vi "products.vi"(8 "error in (no error)":errorcluster, 11 "reference in":refnum<class "Project Panels.lvclass">=refnum) -> (0 "error out":errorcluster, 3 "reference out":refnum<class "Project Panels.lvclass">)   [LabVIEW 2015, in "Project Panels.lvclass"]
uses:
  Project Panels.lvclass
  state.ctl
  <vilib>/Utility/miscctls.llb/LVRowAndColumnUnsignedTypeDef.ctl
  SYS/Devices Controller_llb/deviceType.ctl
  <vilib>/Utility/miscctls.llb/LVRowAndColumnTypeDef.ctl
  SYS/Devices Controller_llb/Devices Controller.lvclass
panel:
  out "title":string="Cosmed Asia Pacific - Products in Aussie"
  in  "tables":T1(tab)
  out "K5":string[][](table)=[["705001", "not active", "K4b2", "not active", "not active", "not active", "not active", "not active", "not active", "not active", "not active", "not active", ""], ["803033", "not active", "K4b2", "not active", "not active", "not active", "not active", "not active", "not active", "not active", "not active", "not active", ""], ["804042", "not active", "K4b2", "not active", "not active", "not active", "not active", "not active", "not active", "not active", "not active", "not active", ""], ["804046", "", "K4b2", "Univ. of Queensland", "St Lucia, Brisbane", "Gary Wilson", "seant@hms.uq.edu.au", "Bellamby", "sep-06", "Italy", "sep-07", "not active", ""], ["804047", "not active", "K4b2", "not active", "not active", "not active", "not active", "not active", "not active", "not active", "not active", "not active", ""], ["9806059", "6.2", "K4b2", "not active", "not active", "not active", "not active", "not active", "not active", "not active", "not active", "not active", ""], ["9806062", "5.1", "K4b2", "Queensland Academy of Sport", "Sunnybank", "Mark Andrews", "mark.andrews@srq.qld.com.au", "Nahtan, GC", "june 2013 in italy for CO2 refurbish", "Italy service", "jun-14", "", ""], ["9807077", "6.0a", "K4b2", "Uni of Canterbury", "Uni of Canterbury", "Gavin Blackwell", "gavin.blackwell@canterbury.ac.nz", "Christchurch", "feb-13", "fede", "feb-14", "", ""], ["9810080", "", "K4b2", "Royal Children's Hospital", "Herston", "Teresa Phillips", "Teresa_Phillips@health.qld.gov.au", "Herston", "jun-06", "Italy", "jun-07", "9/17/2013", ""], ["9903123", "7.2", "K4b2", "Uni of Adelaide", "Uni of Adelaide", "David Bentley", "david.bentley@adelaide.edu.au", "Adelaide", "dic-12", "Serv Italy +valve", "dic-13", "", ""], ["9912206", "7.3", "K4b2", "Uni of Canterbury", "Uni of Canterbury", "Gavin Blackwell", "gavin.blackwell@canterbury.ac.nz", "Christchurch", "feb-13", "fede", "feb-14", "", ""], ["200104325", "8", "K4b2", "Uni of South Australia", "Sansom Institute", "Michelle N. McDonnell", "", "Adelaide", "nov-11", "fede", "dic-12", "9/9/2013", ""], ["200201385", "9.1b", "K4b2", "University of Sydney", "Lidcombe Campus", "Hui Yin Ler  (PhD)", "", "Sydney", "oct-11", "fede", "oct-12", "9/9/2013", ""], ["200205419", "8.0", "K4b2", "University of Sydney", "Liverpool hospital", "Leanne Hassett", "leanne.hassett@sydney.edu.au", "Sydney", "nov-11", "fede", "nov-12", "Not Using in this moment", ""], ["200205423", "9.1b", "K4b2", "University of Sydney", "Lidcombe Campus", "Martin Thomson", "", "Sydney", "feb-10", "italy", "feb-11", "9/9/2013", ""], ["200205424", "7.3", "K4b2", "University of Sydney", "Lidcombe Campus", "Martin Thomson", "", "Sydney", "sep-08", "Italy", "sep-09", "9/10/2013", ""], ["200404607", "", "K4b2", "The Sydney Children's Hospital Network", "Westmead", "Leanne Purcell", "leanne.purcell@health.nsw.gov.au", "Westmead", "nov-08", "italy", "nov-09", "9/17/2013", "Yes, but waiting the start of the testing"], ["200512701", "8.0b", "K4b2", "James Cook Uni", "James Cook Uni", "Anthony Leight", "Anthony.Leicht@jcu.edu.au", "Townsville", "jan-13", "", "jan-14", "", ""], ["200601705", "", "K4b2", "Latrobe University", "Bundoora (Melb)", "Paul Moon", "P.Moon@latrobe.edu.au", "Melbourne", "jan-08", "Italy", "jan-09", "9/17/2013", ""], ["200607745", "", "K4b2", "QUT Brisbane", "Kelvin Grove", "Pei Cher", "pei.cher@qut.edu.au", "BBN", "may-13", "fede", "may-14", "", ""], ["200710813", "", "K4b2", "Victoria Uni", "", "Jessica Meilak", "jessica.meilak@vu.edu.au", "Melb", "jan-12", "Brad", "jan-14", "15/01/14", ""], ["200907909", "9.1b", "K4b2", "Uni of New South Wales", "Uni of New South Wales", "Stephen Redmond", "s.redmond@unsw.edu.au", "Sydney", "sep-12", "fede", "sep-13", "9/17/2013", ""], ["200909916", "", "K4b2", "Uni of Canterbury", "Uni of Canterbury", "Gavin Blackwell", "gavin.blackwell@canterbury.ac.nz", "Christchurch", "feb-13", "fede", "feb-14", "", ""], ["201007964", "", "K4b2", "University of Canberra", "Canberra", "Ben Rattray", "ben.rattray@canberra.edu.au", "Canberra", "mar-12", "", "mar-13", "9/17/2013", ""], ["201009980", "9.1b", "K4b2", "Uni of Technology Sydney", "UTS City Campus", "Steven Su", "steven.su@eng.uts.edu.au", "Sydney", "oct-12", "Medtel (also Lee Valve)", "oct-13", "9/17/2013", ""], ["2011121063", "", "K4b2", "Victoria Uni", "", "Jessica Meilak", "jessica.meilak@vu.edu.au", "Melb", "jan-12", "Brad", "jan-14", "", ""], ["2011121064", "", "K4b2", "Victoria Uni", "", "Jessica Meilak", "jessica.meilak@vu.edu.au", "Melb", "jan-12", "Brad", "jan-14", "", ""], ["2012021076", "", "K4b2", "Demo Unit", "Demo Unit", "TBD", "", "TBD", "sep-13", "Manu-AUS", "sep-14", "", ""], ["2012021080", "", "K4b2", "Massey Univ.", "Wellington", "Brandon Woolley", "B.Woolley@massey.ac.nz", "Wellington", "nov-13", "Manu-AUS", "nov-14", "", ""], ["2012061109", "", "K4b2", "Griffith University Gold Coast Campus", "Gold Coast", "Anna Boehm", "a.boehm@griffith.edu.au", "Gold Coast", "jul-13", "fede", "jul-14", "", ""], ["2012061115", "10.0d", "K4b2", "University of Newcastle", "Callaghan", "Robin Callister", "Robin.Callister@newcastle.edu.au", "Ourimbah", "nov-13", "Manu-AUS", "nov-14", "", ""], ["2012111144", "10.0d", "K4b2", "University of Newcastle", "Callaghan", "Robin Callister", "Robin.Callister@newcastle.edu.au", "Ourimbah", "nov-13", "Manu-AUS", "nov-14", "", ""], ["2012111148", "", "K4b2", "University of Western Sydney", "PENRITH", "Tara Hamilton", "t.hamilton@uws.edu.au", "PENRITH", "dec-13", "Manu-AUS", "dec-14", "", ""], ["2013011158", "10.0d", "K4b2", "University of the Sunshine Coast", "Maroochydore DC", "Ava Kerr", "akerr@usc.edu.au", "Sippy Downs", "may-13", "new", "may-14", "", ""], ["2013031168", "10.0d", "K4b2", "Australian Catholic University", "Sydney", "Phillip Chapman", "Phillip.Chapman@acu.edu.au", "Sydney", "apr-13", "new", "apr-14", "", ""], ["Prova", "", "Prova", "", "", "", "", "", "", "", "", "", ""]]
  out "k4b2":string[][](table)=[["705001", "not active", "K4b2", "not active", "not active", "not active", "not active", "not active", "not active", "not active", "not active", "not active", ""], ["803033", "not active", "K4b2", "not active", "not active", "not active", "not active", "not active", "not active", "not active", "not active", "not active", ""], ["804042", "not active", "K4b2", "not active", "not active", "not active", "not active", "not active", "not active", "not active", "not active", "not active", ""], ["804046", "", "K4b2", "Univ. of Queensland", "St Lucia, Brisbane", "Gary Wilson", "seant@hms.uq.edu.au", "Bellamby", "sep-06", "Italy", "sep-07", "not active", ""], ["804047", "not active", "K4b2", "not active", "not active", "not active", "not active", "not active", "not active", "not active", "not active", "not active", ""], ["9806059", "6.2", "K4b2", "not active", "not active", "not active", "not active", "not active", "not active", "not active", "not active", "not active", ""], ["9806062", "5.1", "K4b2", "Queensland Academy of Sport", "Sunnybank", "Mark Andrews", "mark.andrews@srq.qld.com.au", "Nahtan, GC", "june 2013 in italy for CO2 refurbish", "Italy service", "jun-14", "", ""], ["9807077", "6.0a", "K4b2", "Uni of Canterbury", "Uni of Canterbury", "Gavin Blackwell", "gavin.blackwell@canterbury.ac.nz", "Christchurch", "feb-13", "fede", "feb-14", "", ""], ["9810080", "", "K4b2", "Royal Children's Hospital", "Herston", "Teresa Phillips", "Teresa_Phillips@health.qld.gov.au", "Herston", "jun-06", "Italy", "jun-07", "9/17/2013", ""], ["9903123", "7.2", "K4b2", "Uni of Adelaide", "Uni of Adelaide", "David Bentley", "david.bentley@adelaide.edu.au", "Adelaide", "dic-12", "Serv Italy +valve", "dic-13", "", ""], ["9912206", "7.3", "K4b2", "Uni of Canterbury", "Uni of Canterbury", "Gavin Blackwell", "gavin.blackwell@canterbury.ac.nz", "Christchurch", "feb-13", "fede", "feb-14", "", ""], ["200104325", "8", "K4b2", "Uni of South Australia", "Sansom Institute", "Michelle N. McDonnell", "", "Adelaide", "nov-11", "fede", "dic-12", "9/9/2013", ""], ["200201385", "9.1b", "K4b2", "University of Sydney", "Lidcombe Campus", "Hui Yin Ler  (PhD)", "", "Sydney", "oct-11", "fede", "oct-12", "9/9/2013", ""], ["200205419", "8.0", "K4b2", "University of Sydney", "Liverpool hospital", "Leanne Hassett", "leanne.hassett@sydney.edu.au", "Sydney", "nov-11", "fede", "nov-12", "Not Using in this moment", ""], ["200205423", "9.1b", "K4b2", "University of Sydney", "Lidcombe Campus", "Martin Thomson", "", "Sydney", "feb-10", "italy", "feb-11", "9/9/2013", ""], ["200205424", "7.3", "K4b2", "University of Sydney", "Lidcombe Campus", "Martin Thomson", "", "Sydney", "sep-08", "Italy", "sep-09", "9/10/2013", ""], ["200404607", "", "K4b2", "The Sydney Children's Hospital Network", "Westmead", "Leanne Purcell", "leanne.purcell@health.nsw.gov.au", "Westmead", "nov-08", "italy", "nov-09", "9/17/2013", "Yes, but waiting the start of the testing"], ["200512701", "8.0b", "K4b2", "James Cook Uni", "James Cook Uni", "Anthony Leight", "Anthony.Leicht@jcu.edu.au", "Townsville", "jan-13", "", "jan-14", "", ""], ["200601705", "", "K4b2", "Latrobe University", "Bundoora (Melb)", "Paul Moon", "P.Moon@latrobe.edu.au", "Melbourne", "jan-08", "Italy", "jan-09", "9/17/2013", ""], ["200607745", "", "K4b2", "QUT Brisbane", "Kelvin Grove", "Pei Cher", "pei.cher@qut.edu.au", "BBN", "may-13", "fede", "may-14", "", ""], ["200710813", "", "K4b2", "Victoria Uni", "", "Jessica Meilak", "jessica.meilak@vu.edu.au", "Melb", "jan-12", "Brad", "jan-14", "15/01/14", ""], ["200907909", "9.1b", "K4b2", "Uni of New South Wales", "Uni of New South Wales", "Stephen Redmond", "s.redmond@unsw.edu.au", "Sydney", "sep-12", "fede", "sep-13", "9/17/2013", ""], ["200909916", "", "K4b2", "Uni of Canterbury", "Uni of Canterbury", "Gavin Blackwell", "gavin.blackwell@canterbury.ac.nz", "Christchurch", "feb-13", "fede", "feb-14", "", ""], ["201007964", "", "K4b2", "University of Canberra", "Canberra", "Ben Rattray", "ben.rattray@canberra.edu.au", "Canberra", "mar-12", "", "mar-13", "9/17/2013", ""], ["201009980", "9.1b", "K4b2", "Uni of Technology Sydney", "UTS City Campus", "Steven Su", "steven.su@eng.uts.edu.au", "Sydney", "oct-12", "Medtel (also Lee Valve)", "oct-13", "9/17/2013", ""], ["2011121063", "", "K4b2", "Victoria Uni", "", "Jessica Meilak", "jessica.meilak@vu.edu.au", "Melb", "jan-12", "Brad", "jan-14", "", ""], ["2011121064", "", "K4b2", "Victoria Uni", "", "Jessica Meilak", "jessica.meilak@vu.edu.au", "Melb", "jan-12", "Brad", "jan-14", "", ""], ["2012021076", "", "K4b2", "Demo Unit", "Demo Unit", "TBD", "", "TBD", "sep-13", "Manu-AUS", "sep-14", "", ""], ["2012021080", "", "K4b2", "Massey Univ.", "Wellington", "Brandon Woolley", "B.Woolley@massey.ac.nz", "Wellington", "nov-13", "Manu-AUS", "nov-14", "", ""], ["2012061109", "", "K4b2", "Griffith University Gold Coast Campus", "Gold Coast", "Anna Boehm", "a.boehm@griffith.edu.au", "Gold Coast", "jul-13", "fede", "jul-14", "", ""], ["2012061115", "10.0d", "K4b2", "University of Newcastle", "Callaghan", "Robin Callister", "Robin.Callister@newcastle.edu.au", "Ourimbah", "nov-13", "Manu-AUS", "nov-14", "", ""], ["2012111144", "10.0d", "K4b2", "University of Newcastle", "Callaghan", "Robin Callister", "Robin.Callister@newcastle.edu.au", "Ourimbah", "nov-13", "Manu-AUS", "nov-14", "", ""], ["2012111148", "", "K4b2", "University of Western Sydney", "PENRITH", "Tara Hamilton", "t.hamilton@uws.edu.au", "PENRITH", "dec-13", "Manu-AUS", "dec-14", "", ""], ["2013011158", "10.0d", "K4b2", "University of the Sunshine Coast", "Maroochydore DC", "Ava Kerr", "akerr@usc.edu.au", "Sippy Downs", "may-13", "new", "may-14", "", ""], ["2013031168", "10.0d", "K4b2", "Australian Catholic University", "Sydney", "Phillip Chapman", "Phillip.Chapman@acu.edu.au", "Sydney", "apr-13", "new", "apr-14", "", ""], ["Prova", "", "Prova", "", "", "", "", "", "", "", "", "", ""]]
  out "fitmate":string[][](table)=[["2005090013", "2.2", "Fitmate Pro", "Wesley Weight Management", "Milton", "Liz Ernst", "eernst@lifeshape.com.au", "Milton", "27/09", ""], ["2006020058", "1", "Fitmate WM", "Toombul Medical Centre", "Spring Hill", "Zoe Glover", "toombulmc@gmail.com", "Spring Hill", "27/09", ""], ["2006020059", "1", "Fitmate WM", "RMIT Univ.", "Melbourne", "George Lenon", "george.lenon@rmit.edu.au", "Melbourne", "27/09", ""], ["2006020060", "1", "Fitmate WM", "Logan Hospital", "Meadowbrook", "??", "??", "Meadowbrook", "", ""], ["2006020061", "1.6", "Fitmate WM", "Biomedex (Aust) Pty Ltd", "Woonona", "Biomedex (Aust) Pty Ltd", "??", "Woonona", "", ""], ["2006020077", "1", "Fitmate Pro", "Wesley Weight Management", "Southport", "Sally Jordan", "SJordan@weshealth.com.au", "Southport", "27/09 mail come back / no problem", ""], ["2006020078", "1", "Fitmate Pro", "Life4Ever Pty Ltd", "Arundel", "Michael Tait", "mail@drmichaeltait.com", "Arundel", "27/09 mail come back", ""], ["2006030062", "2.2", "Fitmate WM", "Biomedex (Aust) Pty Ltd", "Woonona", "Biomedex (Aust) Pty Ltd", "??", "Woonona", "", ""], ["2006030083", "2", "Fitmate Pro", "Australian College of Physical Education", "Olympic Park Sydney", "Sven Rees", "srees@acpe.edu.au", "Olympic Park Sydney", "30/09", ""], ["2006030084", "2.3", "Fitmate Pro", "Monash Univ. The Alfred Centre", "Frankston", "Tim Wallace", "tim.wallace@monash.edu", "Frankston", "Case Opned for Macro error", ""], ["2006030085", "2.2", "Fitmate Pro", "Southside Exercise Therapy", "Gymea", "Luke Delvecchio", "southsidepty@optusnet.com.au", "Gymea", "30/09", ""], ["2006060076", "1.1", "Fitmate WM", "Edith Cowan Univ.", "Joondalup", "Amanda Devine", "a.devine@ecu.edu.au", "Joondalup", "30/09", ""], ["2006060078", "1.1", "Fitmate WM", "Edith Cowan Univ.", "Joondalup", "Amanda Devine", "a.devine@ecu.edu.au", "Joondalup", "30/09", ""], ["2006060080", "2.3", "Fitmate WM", "WESLEY Corporate Health", "Brisbane", "Liz Ernst", "eernst@lifeshape.com.au", "Brisbane", "27/09", ""], ["2006080185", "1.1", "Fitmate Pro", "Edith Cowan Univ.", "Joondalup", "Doreen Mackie", "DMackie@hotmail.com", "Joondalup", "Waiting for details from email (n.vrdoljak@ecu.edu.au   )", ""], ["2006080186", "1.1", "Fitmate Pro", "Neocardia PTY LTD", "Noosaville", "Neavison", "Neavison@hotmail.com", "Noosaville", "30/09", ""], ["2006080187", "1.1", "Fitmate Pro", "Kams Health and Fitness", "Armidale", "Kamahl Barhoush", "info@kams.com.au", "Armidale", "doesn't answer/call again", ""], ["2006080188", "1.1", "Fitmate Pro", "Edith Cowan Univ.", "Joondalup", "Doreen Mackie", "DMackie@hotmail.com", "Joondalup", "Waiting for details from email (n.vrdoljak@ecu.edu.au   )", ""], ["2006080189", "1.1", "Fitmate Pro", "Get Back On Track", "Victoria", "Lisa Ham", "LisaH@bigpond.com.au", "Victoria", "doesn't answer/call again", ""], ["2006080190", "1.1", "Fitmate Pro", "Edith Cowan Univ.", "Joondalup", "Doreen Mackie", "DMackie@hotmail.com", "Joondalup", "Waiting for details from email (n.vrdoljak@ecu.edu.au   )", ""], ["2006080191", "1.1", "Fitmate Pro", "One Life", "PADDINGTON", "Justin Lang", "admin@onelifeliveit.net.au", "PADDINGTON", "01/10", "NOT ACTIVE"], ["2007030363", "1.1", "Fitmate Pro", "X-Fitness Systems Ltd", "Auckland,", "Scott Tibbutt", "scott@xfitness.co.nz", "Auckland,", "30/09", ""], ["2007030372", "1.1", "Fitmate Pro", "Edith Cowan Univ.", "Joondalup", "Doreen Mackie", "DMackie@hotmail.com", "Joondalup", "Waiting for details from email (n.vrdoljak@ecu.edu.au   )", ""], ["2007030373", "1.1", "Fitmate Pro", "Edith Cowan Univ.", "Joondalup", "Doreen Mackie", "DMackie@hotmail.com", "Joondalup", "Waiting for details from email (n.vrdoljak@ecu.edu.au   )", ""], ["2007030375", "1.1", "Fitmate Pro", "Vision Health and Fitness", "Toowoomba", "Troy Taylor", "troy@visionhealth.com.au", "Toowoomba", "30/09", ""], ["2007050155", "2", "Fitmate WM", "Fitness Fusion", "Ohope", "Erin Baker", "paul@fitnessfusion.co.nz", "Ohope", "30/09", ""], ["2007050156", "1.1", "Fitmate WM", "X-Fitness Systems Ltd", "Auckland,", "X-Fitness Systems Ltd", "jeremyu@uhl.co.nz", "Auckland,", "30/09", ""], ["2007050157", "2.2", "Fitmate WM", "Wesley Weight Management", "Milton", "Liz Ernst", "eernst@lifeshape.com.au", "Milton", "27/09", ""], ["2007050158", "2.2", "Fitmate WM", "WESLEY Corporate Health", "Brisbane", "Liz Ernst", "eernst@lifeshape.com.au", "Brisbane", "27/09", ""], ["2007050159", "1.1", "Fitmate WM", "Wesley Weight Management", "Rockhampton", "Simon Fawssett", "sfawssett@weshealth.com.au", "Rockhampton", "no problem", ""], ["2007050160", "2.2", "Fitmate WM", "WESLEY Corporate Health", "Brisbane", "Liz Ernst", "eernst@lifeshape.com.au", "Brisbane", "27/09", ""], ["2007050161", "1.1", "Fitmate WM", "Pyrmont Health & Fitness Club", "Pyrmont", "Antoine Poulter", "??", "Pyrmont", "", ""], ["2007050376", "1.1", "Fitmate Pro", "Edith Cowan Univ.", "Joondalup", "Doreen Mackie", "DMackie@hotmail.com", "Joondalup", "Waiting for details from email (n.vrdoljak@ecu.edu.au   )", ""], ["2007050377", "1.1", "Fitmate Pro", "Elgin Street Medical Centre", "Carlton", "Daniel Cobb", "dcobb@live.com.au", "Carlton", "30/09", ""], ["2007050378", "1.1", "Fitmate Pro", "Pyrmont Health & Fitness Club", "Pyrmont", "Justine Justine", "??", "Pyrmont", "", ""], ["2007050379", "1.6", "Fitmate Pro", "HERT", "Millers Point", "Mark Newton", "mark@hert.com.au", "Millers Point", "30/09", ""], ["2007050380", "1.1", "Fitmate Pro", "Edith Cowan Univ.", "Joondalup", "Doreen Mackie", "DMackie@hotmail.com", "Joondalup", "Waiting for details from email (n.vrdoljak@ecu.edu.au   )", ""], ["2007050381", "1.6", "Fitmate Pro", "Fitness Development Australia", "Sydney", "Fitness Development Australia", "zarko_mikulic@hotmail.com", "Sydney", "30/09", ""], ["2007050388", "1.1", "Fitmate Pro", "ULO Pty Ltd", "Roebourne Court", "Adam Brown", "adam@ulo.com.au", "Daisy Hill", "30/09", ""], ["2007050395", "1.6", "Fitmate Pro", "Biomedex (Aust) Pty Ltd", "Woonona", "Biomedex (Aust) Pty Ltd", "??", "Woonona", "", ""], ["2007050404", "1.1", "Fitmate Pro", "Biomedex (Aust) Pty Ltd", "Woonona", "Biomedex (Aust) Pty Ltd", "??", "Woonona", "", ""], ["2007060413", "2", "Fitmate Pro", "Biomedex (Aust) Pty Ltd", "Woonona", "Biomedex (Aust) Pty Ltd", "??", "Woonona", "", ""], ["2007060415", "1.1", "Fitmate Pro", "Mater Childrens Hospital", "South Brisbane", "Gary Leong", "gary.leong@mater.org.au", "South Brisbane", "1/10/2013", ""], ["2007060417", "1.1", "Fitmate Pro", "Ray Kelly Fitness", "Blacktown", "Ray Kelly", "maxvel01@hotmail.com", "Blacktown", "30/09", ""], ["2007100277", "2.2", "Fitmate WM", "Biomedex (Aust) Pty Ltd", "Woonona", "Biomedex (Aust) Pty Ltd", "??", "Woonona", "", ""], ["2007100278", "1.1", "Fitmate WM", "Tone Up Weight Loss", "Campbelltown", "Christopher Satara", "scott@swphysio.com.au'", "Campbelltown", "08/10", ""], ["2007100279", "1.6", "Fitmate WM", "Biomedex (Aust) Pty Ltd", "Woonona", "Biomedex (Aust) Pty Ltd", "??", "Woonona", "", ""], ["2007100281", "2.2", "Fitmate WM", "Biomedex (Aust) Pty Ltd", "Woonona", "Biomedex (Aust) Pty Ltd", "??", "Woonona", "", ""], ["2007100282", "2.2", "Fitmate WM", "Biomedex (Aust) Pty Ltd", "Woonona", "Biomedex (Aust) Pty Ltd", "??", "Woonona", "", ""], ["2007100484", "2.3", "Fitmate Pro", "Univ. of Auckland", "Auckland", "Grant Mawston", "", "Auckland", "", ""], ["2008010568", "2.3", "Fitmate Pro", "Australian College of", "Olympic Park Sydney", "Sven Rees", "srees@acpe.edu.au", "Olympic Park Sydney", "30/09", ""], ["2008010576", "2.2", "Fitmate Pro", "Body Dynamics Illawarra", "Bulli", "Alan Wilkie", "alan@bodydynamics.com.au", "Bulli", "01/10", ""], ["2008010578", "2.2", "Fitmate Pro", "Cardiofirst Pty Ltd.", "Frenchs Forest", "Camilla", "reports@cardiofirst.com.au", "Frenchs Forest", "", ""], ["2008010579", "2.2", "Fitmate Pro", "Biomedex (Aust) Pty Ltd", "Woonona", "Biomedex (Aust) Pty Ltd", "??", "Woonona", "", ""], ["2008010585", "1.1", "Fitmate Pro", "Biomedex (Aust) Pty Ltd", "Woonona", "Biomedex (Aust) Pty Ltd", "??", "Woonona", "", ""], ["2008030035", "1.6", "Fitmate MED", "Biomedex (Aust) Pty Ltd", "Woonona", "Biomedex (Aust) Pty Ltd", "??", "Woonona", "", ""], ["2008030037", "2", "Fitmate MED", "Biomedex (Aust) Pty Ltd", "Woonona", "Biomedex (Aust) Pty Ltd", "??", "Woonona", "", ""], ["2008040639", "1.5", "Fitmate Pro", "", "Wellington", "Stefan Darrall", "stefan.darrall@xtra.co.nz", "Wellington", "01/10", ""], ["2008040645", "2,2", "Fitmate Pro", "FEDERICO ZANELLA", "Narrabeen", "Federico Zanella", "", "Narrabeen", "", ""], ["2008090067", "2", "Fitmate MED", "Biomedex Pty Ltd.", "Bellambi", "Biomedex Pty Ltd.", "??", "Bellambi", "", ""], ["2008090071", "2", "Fitmate MED", "Logan City Council", "Logan Central", "Campbell MacGregor (not work there anymore)", "council@logan.qld.gov.au", "Logan Central", "08/10 request info sent", ""], ["2008090073", "1.6", "Fitmate MED", "Biomedex (Aust) Pty Ltd", "Woonona", "Biomedex (Aust) Pty Ltd", "??", "Woonona", "", ""], ["2008090075", "1.6", "Fitmate MED", "Enriched Health and Fizzsport Physiotherapy", "Port Macquarie", "Simon Turnball", "simon.turnbull@enrichedhealth.com.au", "Port Macquarie", "01/10", ""], ["2008090076", "2", "Fitmate MED", "Biomedex Pty Ltd.", "Bellambi", "Biomedex Pty Ltd.", "??", "Bellambi", "", ""], ["2008100402", "1.6", "Fitmate WM", "LSNDS P/L", "Mount Eliza", "Andrew Harland", "lsnds@optusenet.com.au", "Mount Eliza", "", ""], ["2008100403", "2.2", "Fitmate WM", "Monash Univ. The Alfred Centre", "Melbourne", "Emma Ridley", "emma.ridley@monash.edu", "Melbourne", "01/10", ""], ["2008100404", "1.6", "Fitmate WM", "The Prince Charles Hospital", "Brisbane", "Renee Rogers", "", "Brisbane", "", ""], ["2008100405", "2.2", "Fitmate WM", "Monash Univ. The Alfred Centre", "Melbourne", "Emma Ridley", "emma.ridley@monash.edu", "Melbourne", "01/10", ""], ["2008100408", "1.6", "Fitmate WM", "Univ. of Newcastle (AUSTRALIA)", "Tamworth", "Leanne Brown", "leanne.brown@newcastle.edu.au", "Tamworth", "01/10", ""], ["2009070009", "1,6", "Fitmate Pro", "Ray Kelly Fitness", "Blacktown", "Ray Kelly", "maxvel01@hotmail.com", "Blacktown", "30/09", ""], ["2010011057", "2", "Fitmate Pro", "Swift Sports Performance Equip", "Lismore", "Mark Fisher", "mark@spe.com.au", "Lismore", "01/10", ""], ["2010021097", "2", "Fitmate Pro", "ASCENCIA Pty. Limited", "Notting Hill", "Michael Panagopoulos", "michael@ascencia.com.au", "Notting Hill", "", ""], ["2010021098", "2", "Fitmate Pro", "Melbourne Sports & Allied Health Clinic", "Essendon North", "Simon Sostaric", "simon@msahc.com.au", "Essendon North", "01/10", ""], ["2010041123", "2", "Fitmate Pro", "Pymble Ladies College", "Pymble", "Thomas Kindred", "tkindred@pymblelc.nsw.edu.au", "Pymble", "01/10", ""], ["2010041133", "2", "Fitmate Pro", "New Zealand Institute of Sport", "Wellington", "Tony Rogers", "tony.r@nzis.co.nz", "Wellington", "info da fede", ""], ["2010091200", "2", "Fitmate Pro", "Univ. of Western Sydney", "Sydney", "Andrew Webber", "a.webber@uws.edu.au / a.boros@uws.edu.au", "Sydney", "01/10", ""], ["2010091208", "2.2", "Fitmate Pro", "AusFitness Test", "Burleigh Heads", "Daniel Mckenzie", "dan@ausfitnesstest.com", "Burleigh Heads", "01/10", ""], ["2010111079", "2", "Fitmate MED", "Xceler8", "Wagga", "Kerry Podmore", "Kerry-xceler8@bigpond.com", "Wagga", "01/10", ""], ["2010121080", "2", "Fitmate MED", "", "Toormina, Boambee", "Chris Cherry", "", "Toormina, Boambee", "", ""], ["2010121084", "2", "Fitmate MED", "Victoria University", "St.ALbans", "Christos Stathis", "christos.stathis@vu.edu.au", "St.ALbans", "01/10", ""], ["2010121085", "2", "Fitmate MED", "Victoria University", "St.ALbans", "Christos Stathis", "christos.stathis@vu.edu.au", "St.ALbans", "01/10", ""], ["2010121088", "2", "Fitmate MED", "", "Melbourne Nth.", "T. Goh", "??", "Melbourne Nth.", "", ""], ["2010121250", "2.2", "Fitmate Pro", "Otago Polytechnic", "Dunedin", "Hayden Croft", "Hayden.Croft@op.ac.nz", "Dunedin", "01/10", ""], ["2011021095", "2", "Fitmate MED", "CHM Management", "South Melbourne", "Kirsty Lerm", "klerm@chm.com.au", "South Melbourne", "01/10", ""], ["2011041238", "2.2", "Fitmate WM", "University of the Sunshine Coast", "Sippy Downs", "Gary Slater", "gslater@usc.edu.au", "Maroochydore DC", "01/10", "accepted 04/10"], ["2011061360", "2.2", "Fitmate Pro", "Sports Orthopaedic and Rehabilitation", "Sydney", "Peter McDonald", "pmcdfitness@gmail.com.au'", "Sydney", "", ""], ["2011061363", "2.2", "Fitmate Pro", "Sports Orthopaedic and Rehabilitation", "Sydney", "Peter McDonald", "pmcdfitness@gmail.com.au'", "Sydney", "", ""], ["2011071270", "2.2", "Fitmate WM", "University of Otago", "Dunedin", "Gavin Hendry", "gavin.hendry@otago.ac.nz", "Dunedin", "01/10", ""], ["2011111148", "2", "Fitmate MED", "JLM Accutek Health", "Homebush", "Lorrence(Lorenzo) Platania", "??", "Homebush", "", ""], ["2011111155", "2", "Fitmate MED", "JLM Accutek Health", "Homebush", "Lorrence(Lorenzo) Platania", "??", "Homebush", "", ""], ["2011121441", "2.2", "Fitmate Pro", "The Scots College", "Bellevue Hill", "Tenzing Tsewang", "t.tsewang@tsc.nsw.edu.au", "Bellevue Hill", "01/10", ""], ["2011121443", "2.2", "Fitmate Pro", "Sydney Sports & Exercise", "Sydney Olympic Park", "Dean McNamara", "", "Sydney Olympic Park", "", ""], ["2012031327", "2.2", "Fitmate WM", "Univ. of Adelaide", "Adelaide", "Univ. of Adelaide", "", "Adelaide", "", ""], ["2012050009", "2,3", "Fitmate GS", "Belconnen Specialist Center", "Bruce-Canberra", "Mariame Iraki", "", "Bruce-Canberra", "", ""], ["2012061551", "2.2", "Fitmate Pro", "The Scots College", "Bellevue Hill", "Tenzing Tsewang", "t.tsewang@tsc.nsw.edu.au", "Bellevue Hill", "01/10", ""], ["2012061552", "2.2", "Fitmate Pro", "The Scots College", "Bellevue Hill", "Tenzing Tsewang", "t.tsewang@tsc.nsw.edu.au", "Bellevue Hill", "01/10", ""], ["2012061554", "2.2", "Fitmate Pro", "The Scots College", "Bellevue Hill", "Tenzing Tsewang", "t.tsewang@tsc.nsw.edu.au", "Bellevue Hill", "01/10", ""], ["2012091028", "2,3", "Fitmate GS", "The University of Newcastle (AUS)", "Callaghan", "Anna Bukey", "Anna.Bukey@newcastle.edu.au", "Callaghan", "01/10", ""], ["2012101617", "2.3", "Fitmate Pro", "FEDERICO ZANELLA", "Narrabeen", "Federico Zanella", "", "Narrabeen", "", ""], ["2012101619", "2.3", "Fitmate Pro", "Adelaide Exercise Physiology (AEP)", "", "Reuben Vanderzalm", "reuben@aep.net.au", "", "01/10", ""], ["2012111654", "2.2", "Fitmate Pro", "Vascular Ultrasound Partners Pty Ltd", "Adelaide", "Jim Gotting", "emac2403@gmail.com", "Adelaide", "01/10", ""], ["2013011031", "2,3", "Fitmate GS", "FEDERICO ZANELLA", "Narrabeen", "Federico Zanella", "", "Narrabeen", "", ""], ["2013021388", "2.2", "Fitmate WM", "Monash Univ. The Alfred Centre", "Melbourne", "Emma Ridley", "emma.ridley@monash.edu", "Melbourne", "01/10", ""], ["2013041734", "2.2", "Fitmate Pro", "SA Ambulance", "Eastwood", "Adam Zerner", "adam.zerner@health.sa.gov.au", "Eastwood", "01/10", ""], ["2013061753", "2.2", "Fitmate Pro", "James Cook University", "Douglas", "Anthony Leight", "Anthony.Leicht@jcu.edu.au", "Townsville", "01/10", ""], ["20050800003", "1.6", "Fitmate Pro", "Biomedex (Aust) Pty Ltd", "Woonona", "Biomedex (Aust) Pty Ltd", "??", "Woonona", "", ""]]
  out "RMR":string[][](table)=[["2009010042", "", "RMR + ICU", "Monash Univ. The Alfred Centre", "Melbourne", "Emma Ridley", "Emma.Ridley@med.monash.edu.au", "Melbourne", "", ""], ["2010020172", "", "RMR + ICU", "Prince Charles Hospital", "Brisbane", "Vanessa King", "Vanessa_King@health.qld.gov.au", "Brisbane", "", ""], ["2010080174", "", "RMR + ICU", "Monash Univ. The Alfred Centre", "Melbourne", "Emma Ridley", "Emma.Ridley@med.monash.edu.au", "Melbourne", "", ""], ["2010110180", "", "RMR + ICU", "Monash Univ. The Alfred Centre", "Melbourne", "Emma Ridley", "Emma.Ridley@med.monash.edu.au", "Melbourne", "", ""], ["2010110181", "", "RMR + ICU", "Gold Coast Hospital and Robina", "Southport", "Alan Spencer", "alan_spencer@healthqld.gov.au", "Southport", "", ""], ["2011050212", "", "RMR + ICU", "John Hunter Hospital", "New Lambton Heights", "Justin Singleton", "justin.singleton@hnehealth.nsw.gov.au", "New Lambton Heights", "", ""], ["2011110238", "", "RMR", "Royal Prince Alfred Hospital", "Camperdown", "Joanne Heyman", "joanne.heyman@sswahs.nsw.gov.au", "Camperdown", "", ""], ["2012110294", "", "RMR", "University of the Sunshine Coast", "Maroochydore DC", "Gary Slater", "gslater@usc.edu.au", "Maroochydore DC", "", ""], ["2013020316", "", "RMR + ICU", "Royal Perth Hospital", "Perth", "Wayne Epton", "wayne.epton@health.wa.gov.au", "Perth", "", ""], ["2013050335", "", "RMR + ICU", "Gold Coast Hospital and Robina", "Southport", "Alan Spencer", "alan_spencer@healthqld.gov.au", "Southport", "", ""], ["2013050332", "", "RMR", "Auckland City Hospital", "Auckland", "Shay McGuinness", "", "Auckland", "", ""], ["2013050330", "", "RMR + ICU", "University of Queensland", "Herston", "Alexia Murphy", "alexia.murphy@uq.edu.au", "Herston", "", ""]]
  out "CPET":string[][](table)=[["9807035", "5", "Quark b2", "The Royal Melbourne Institute of Technology - RMIT", "Bundoora", "", "", "", "", ""], ["9901046", "", "Quark b2", "Biomedex", "", "", "", "", "", ""], ["9905053", "5.1a", "Quark b2", "Baker Medical Research Institute", "", "", "", "", "", ""], ["200601281", "", "Quark b2", "Ultra Thoroughbred Racing Pty. Ltb", "Green Iris", "Rod Cedaro", "rod.cedaro@gmail.com", "Rod Cedaro", "", ""], ["2007060003", "", "Quark CPET", "Liverpool Hospital", "Liverpool", "Mark Newman", "Mark.Newman@sswahs.nsw.gov.au", "Liverpool", "", ""], ["2008030037", "10.0d", "Quark CPET", "University Otago", "Dunedin", "Nigel Barrett", "nigel.barrett@otago.ac.nz", "Dunedin", "", ""], ["2008030006", "", "Quark PFT/CPET Nutritional", "University Otago", "Dunedin", "Dene Irvine", "dene.irvine@otago.ac.nz", "Dunedin", "", ""], ["2008050039", "9", "Quark CPET", "Victorian Institute of Sport", "Melbourne", "Simon Blundell", "simon.blundell@vis.org.au", "Melbourne", "", ""], ["2008120093", "9.1b", "Quark CPET", "Griffith University Gold Coast Campus", "Gold Coast", "Caroline Young", "caroline.b.young@griffith.edu.au", "Gold Coast", "", ""], ["2009100185", "10.0d", "Quark CPET", "University of Otago", "Dunedin", "Nigel Barrett", "nigel.barrett@otago.ac.nz", "Dunedin", "", ""], ["2010020214", "", "Quark CPET", "Canberra Hospital", "Garran", "Leonard Arnolda", "", "Garran", "", ""], ["2011110397", "10.0d", "Quark CPET", "Univ. of Sydney", "Lidcombe", "Corinne Caillaud", "corinnecalillaud@sidney.edu.au", "Lidcombe", "", ""], ["2011110398", "10.0d", "Quark CPET", "Univ. of Sydney", "Lidcombe", "Corinne Caillaud", "corinnecalillaud@sidney.edu.au", "Lidcombe", "", ""], ["2012020412", "10.0d", "Quark CPET", "University of Otago", "Dunedin", "Nigel Barrett", "nigel.barrett@otago.ac.nz", "Dunedin", "", ""], ["2011120402", "10.0d", "Quark CPET", "The Scots College", "Bellevue Hill", "Tenzing Tsewang", "t.tsewang@tsc.nsw.edu.au", "Bellevue Hill", "", ""], ["2012100477", "10.0d", "Quark CPET", "Victoria University", "Footscray", "Jessica Meilak", "jessica.meilak@vu.edu.au", "Footscray", "", ""], ["2012060085", "10.0d", "Quark CPET", "Victoria University", "Melbourne", "Bradley Gatt", "bradley.gatt@vu.edu.au", "Melbourne", "", ""], ["2012120094", "10.0e", "Quark CPET", "Fede", "DEMO", "DEMO", "DEMO", "DEMO", "", ""], ["2013020524", "", "Quark CPET", "Australian Catholic University - ACU", "Strathfield", "Anoj Poudyal", "anoj.poudyal@acu.edu.au", "Strathfield", "", ""], ["2013060561", "", "Quark CPET", "James Cook University", "Townsville", "Anthony Leight", "Anthony.Leicht@jcu.edu.au", "Douglas", "", ""], ["2013110612", "", "Quark CPET", "Australian Catholic University BBN", "Virginia", "Tim Blackmore", "tim.blackmore@acu.edu.au", "Banyo", "", ""], ["2013120110", "", "Quark CPET", "Australian Catholic University BBN", "Virginia", "Tim Blackmore", "tim.blackmore@acu.edu.au", "Banyo", "", ""]]
  out "BB-PFT":string[][](table)=[["2009010042", "", "RMR + ICU", "Monash Univ. The Alfred Centre", "Melbourne", "Emma Ridley", "Emma.Ridley@med.monash.edu.au", "Melbourne", "", ""], ["2010020172", "", "RMR + ICU", "Prince Charles Hospital", "Brisbane", "Vanessa King", "Vanessa_King@health.qld.gov.au", "Brisbane", "", ""], ["2010080174", "", "RMR + ICU", "Monash Univ. The Alfred Centre", "Melbourne", "Emma Ridley", "Emma.Ridley@med.monash.edu.au", "Melbourne", "", ""], ["2010110180", "", "RMR + ICU", "Monash Univ. The Alfred Centre", "Melbourne", "Emma Ridley", "Emma.Ridley@med.monash.edu.au", "Melbourne", "", ""], ["2010110181", "", "RMR + ICU", "Gold Coast Hospital and Robina", "Southport", "Alan Spencer", "alan_spencer@healthqld.gov.au", "Southport", "", ""], ["2011050212", "", "RMR + ICU", "John Hunter Hospital", "New Lambton Heights", "Justin Singleton", "justin.singleton@hnehealth.nsw.gov.au", "New Lambton Heights", "", ""], ["2011110238", "", "RMR", "Royal Prince Alfred Hospital", "Camperdown", "Joanne Heyman", "joanne.heyman@sswahs.nsw.gov.au", "Camperdown", "", ""], ["2012110294", "", "RMR", "University of the Sunshine Coast", "Maroochydore DC", "Gary Slater", "gslater@usc.edu.au", "Maroochydore DC", "", ""], ["2013020316", "", "RMR + ICU", "Royal Perth Hospital", "Perth", "Wayne Epton", "wayne.epton@health.wa.gov.au", "Perth", "", ""], ["2013050335", "", "RMR + ICU", "Gold Coast Hospital and Robina", "Southport", "Alan Spencer", "alan_spencer@healthqld.gov.au", "Southport", "", ""], ["2013050332", "", "RMR", "Auckland City Hospital", "Auckland", "Shay McGuinness", "", "Auckland", "", ""], ["2013050330", "", "RMR + ICU", "University of Queensland", "Herston", "Alexia Murphy", "alexia.murphy@uq.edu.au", "Herston", "", ""]]
  out "BP":string[][](table)=[["1018", "", "BP GS", "Uni of Adelaide", "Adelaide", "", "", "", "", ""], ["3054", "", "BP DOS", "Uni of Queensland", "Brisbane", "", "", "", "", ""], ["3268", "", "BP DOS W", "Queensland Univ. of Technology", "Kelvin grove", "Rachel Wood", "re.wood@qut.edu.au", "Kelvin grove", "", ""], ["3367", "", "BP W", "Queensland University of Technology", "Kelvin Grove", "Rachel Wood", "re.wood@qut.edu.au", "", "", ""], ["3436", "", "BP W", "Princess Margaret Hospital for Children", "Perth", "David Forbes", "david.forbes@health.wa.gov.au", "Perth", "", ""], ["3529", "5.1.0", "BP GS", "Monash Medical Centre", "Clayton", "Sharon Marks", "sharon@fpds.com.au", "Clayton", "", ""], ["3562", "", "BP GS", "Massey University", "Palmerston North", "Kevin Pedley", "k.c.pedley@massey.ac.nz", "Palmerston North", "", ""], ["3563", "4.2.4", "BP GS", "Bodyology Exercise Science Studio", "Notting Hill", "Andrew Garlick", "andrew@bodyologystudio.com.au", "Notting Hill", "", ""], ["3640", "", "BP GS", "Wesley Research Institute", "Toowong", "Greg Hafner", "ghafner@wesleyresearch.com.au", "Toowong", "", ""], ["3788", "", "BP GS", "Federico", "Federico", "Federico", "", "Federico", "", ""], ["3793", "", "BP GS", "University of the Sunshine Coast", "Maroochydore DC", "Gary Slater", "gslater@usc.edu.au", "Maroochydore DC", "", ""], ["3821", "", "BP GS", "The Scots College", "Bellevue Hill", "Tenzing Tsewang", "t.tsewang@tsc.nsw.edu.au", "Bellevue Hill", "", ""], ["3852", "", "BP GS", "Univ. of Adelaide", "Adelaide", "Univ. of Adelaide", "", "Adelaide", "", ""], ["3868", "5.2.0", "BP GS", "Univ. of Sydney", "Sydney", "Amanda Sainsbury Salis", "amanda.sainsbury-salis@sydney.edu.au", "Sydney", "", ""], ["3930", "", "BP GS", "Paula Serena Pool", "Townsville", "Paula Serena Pool", "", "Townsville", "", ""], ["3947", "", "BP GS", "Paula Serena Pool", "Townsville", "Paula Pool", "", "West End", "", ""], ["3993", "", "BP GS", "Queensland Univ. of Technology", "Kelvin grove", "Nuala Byrne", "n.byrne@qut.edu.au", "Kelvin grove", "", ""], ["4063", "", "BP ST", "Queensland Univ. of Technology", "Kelvin grove", "Rachel Wood", "re.wood@qut.edu.au", "Kelvin grove", "", ""], ["4539", "", "BP EX", "World Gym Ashmore", "Ashmore", "Sarah Friebe", "sarah@worldgymashmore.com.au", "Ashmore", "", ""], ["COSEMD USA 1", "", "BP GS", "University of the Sunshine Coast", "Maroochydore DC Qld", "University of the Sunshine Coast", "", "Maroochydore DC Qld", "", ""]]
  out "PP":string[][](table)=[["6025", "", "PP", "King Edward Memorial", "Perth", "Gemma McLeod", "mcleod.gemma1@gmail.com", "Perth", "", ""], ["6088", "", "PP", "Univ. of Sydney", "Penrith", "Ralph Nanan", "ralph.nanan@sydney.edu.au", "Penrith", "", ""], ["6021", "", "PP", "University of Queensland Centre for Clinical Research", "Herston", "Barbara Lingwood", "b.lingwood@uq.edu.au", "Herston", "", ""], ["6023", "", "PP", "University of Queensland Centre for Clinical Research", "Herston", "Barbara Lingwood", "b.lingwood@uq.edu.au", "Herston", "", ""], ["6082", "", "PP", "Massey Univ.", "Palmerston North", "Jane Coad", "CoadJ.Coad@massey.ac.nz", "Palmerston North", "", ""], ["6044", "", "PP", "Royal Prince Alfred Hospital", "Camperdown", "Emily Bek", "emily.bek@sydney.edu.au", "Camperdown", "", ""]]
  in  "Delete Item":bool
  in  "Send Follow Up":bool
  in  "Search Item":bool
  in  "Edit Item":bool
  in  "New Item":bool
  out "Item Selected (S/N):":string
  out "statuBar":string
  in  "Stop Button":bool
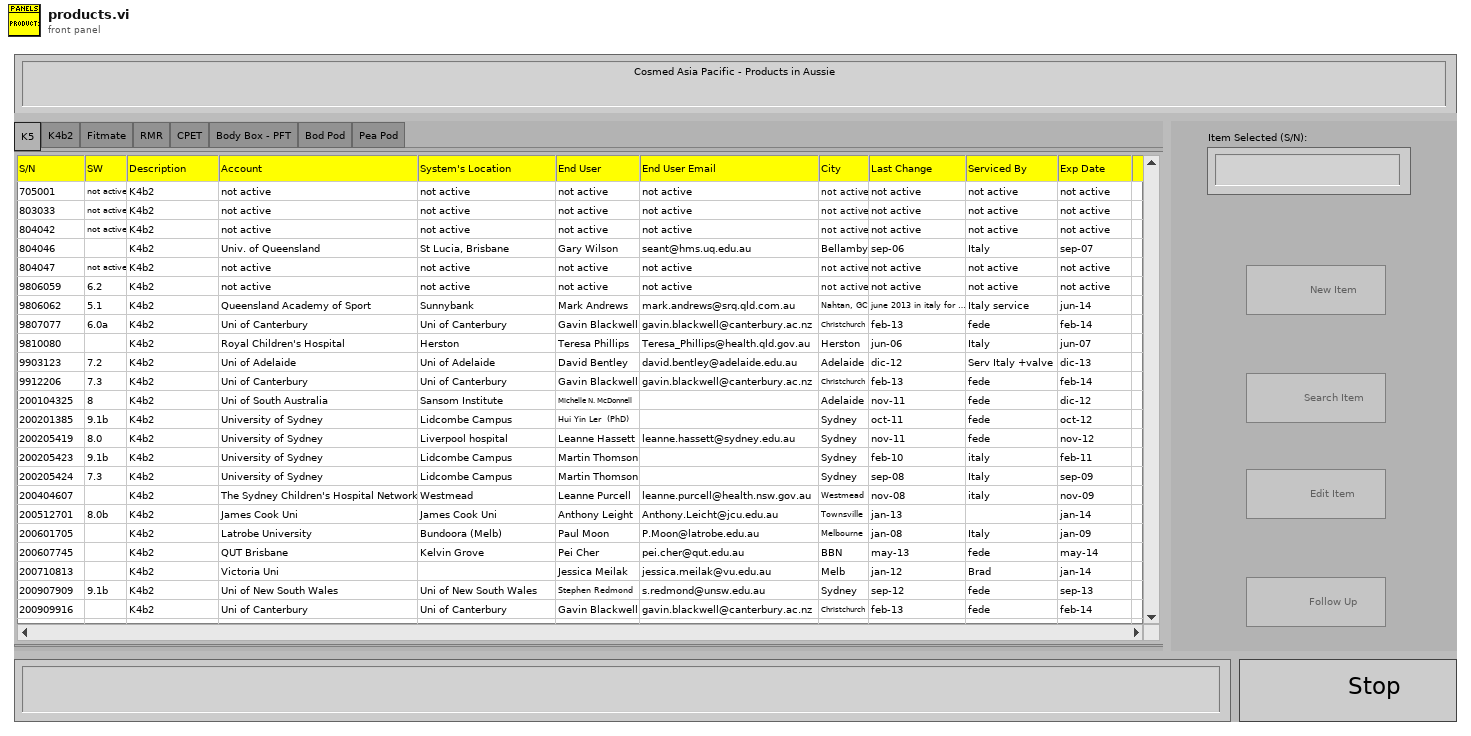
[diagram p1: front panel]
types:
  T1 = enum32{"K5", "K4b2", "Fitmate", "RMR", "CPET", "Body Box - PFT", "Bod Pod", "Pea Pod"}
  T2 = typedef "Project Panels.lvclass/state.ctl" = enum16{"initiate", "waitEvent", "newItem", "searchItem", "editItem", "sendFollowUp", "deleteItem", "stop"}
  T3 = typedef "LVRowAndColumnUnsignedTypeDef.ctl" = cluster{"Row":u32, "Column":u32}
  T4 = enum8{"Enabled", "Disabled", "Disabled and Grayed Out"}
  T5 = typedef "Devices Controller.lvclass/deviceType.ctl" = enum16{"k5", "k4b2", "fitmate", "cpet", "rmr", "bodyBoxPft", "bp", "pp"}
  T6 = typedef "LVRowAndColumnTypeDef.ctl" = cluster{"Row":i32, "Column":i32}
  T7 = typedef "Project Panels.lvclass/ObjectAttributesRef.ctl" = refnum<data-value>
  T8 = typedef "Project Panels.lvclass/ObjectAttributes.ctl" = cluster{"MyAttribute":dbl, "device_controller_ref":refnum<class "Devices Controller.lvclass">, "file_controller_ref":refnum<class "File Controller.lvclass">, "item_controller_ref":refnum<class "Items Controller.lvclass">, "item_tables":cluster{"checkIN":string[][], "checkOUT":string[][], "storage":string[][]}, "quickbook_table":cluster{"notes":string[][]}, "notification_controller_ref":refnum<class "Notification Controller.lvclass">, "partstracking_controller_ref":refnum<class "PartsTracking Controller.lvclass">, "product_tables":cluster{"k4b2":string[][], "fitmate":string[][], "RMR":string[][], "CPET":string[][], "BP":string[][], "PP":string[][], "k5":string[][], "bb-pft":string[][]}, "rowsColour":u32[]}
  T9 = cluster{"k4b2":string[][], "fitmate":string[][], "RMR":string[][], "CPET":string[][], "BP":string[][], "PP":string[][], "k5":string[][], "bb-pft":string[][]}
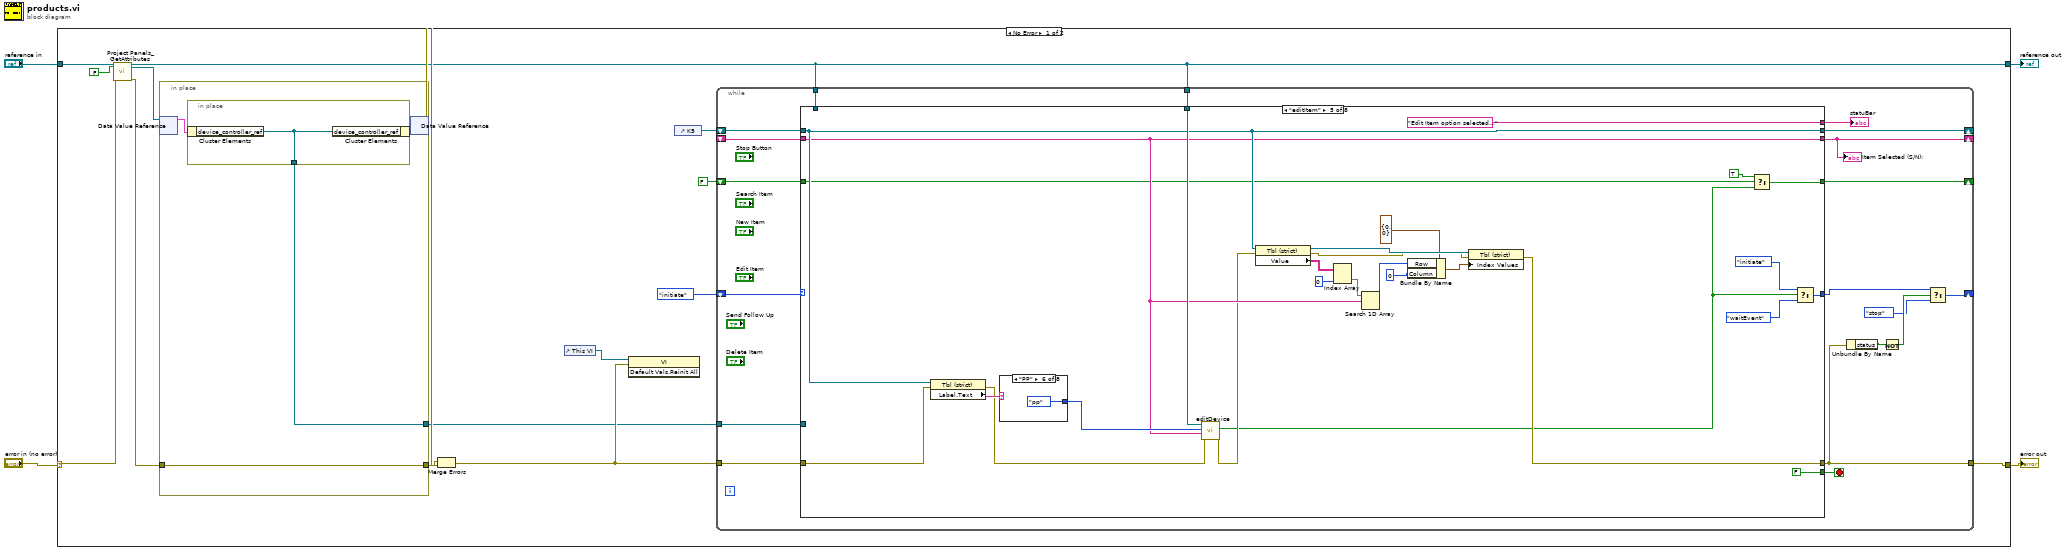
[diagram p0: block diagram]
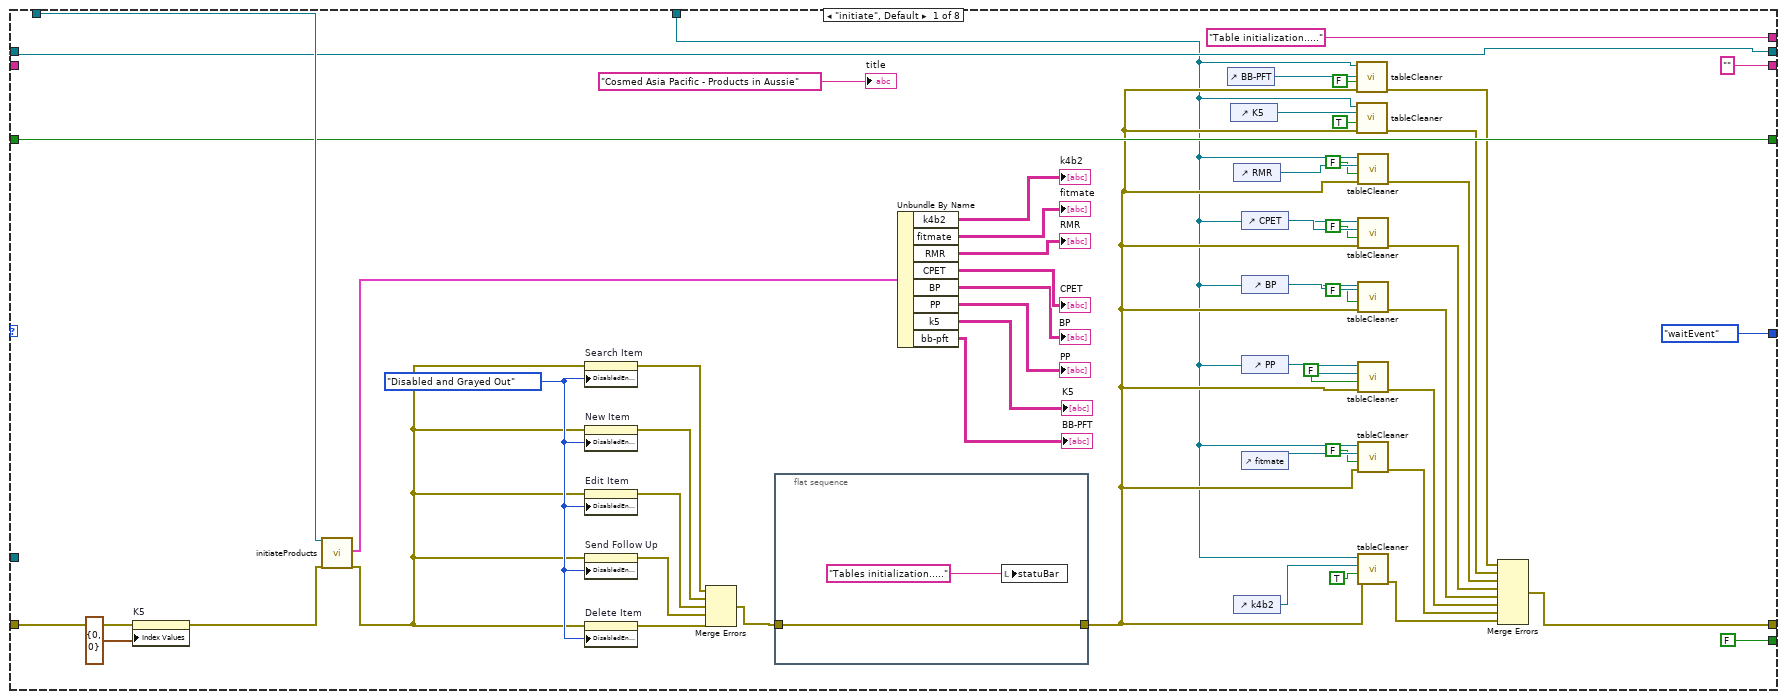
[diagram p2: hidden frame]
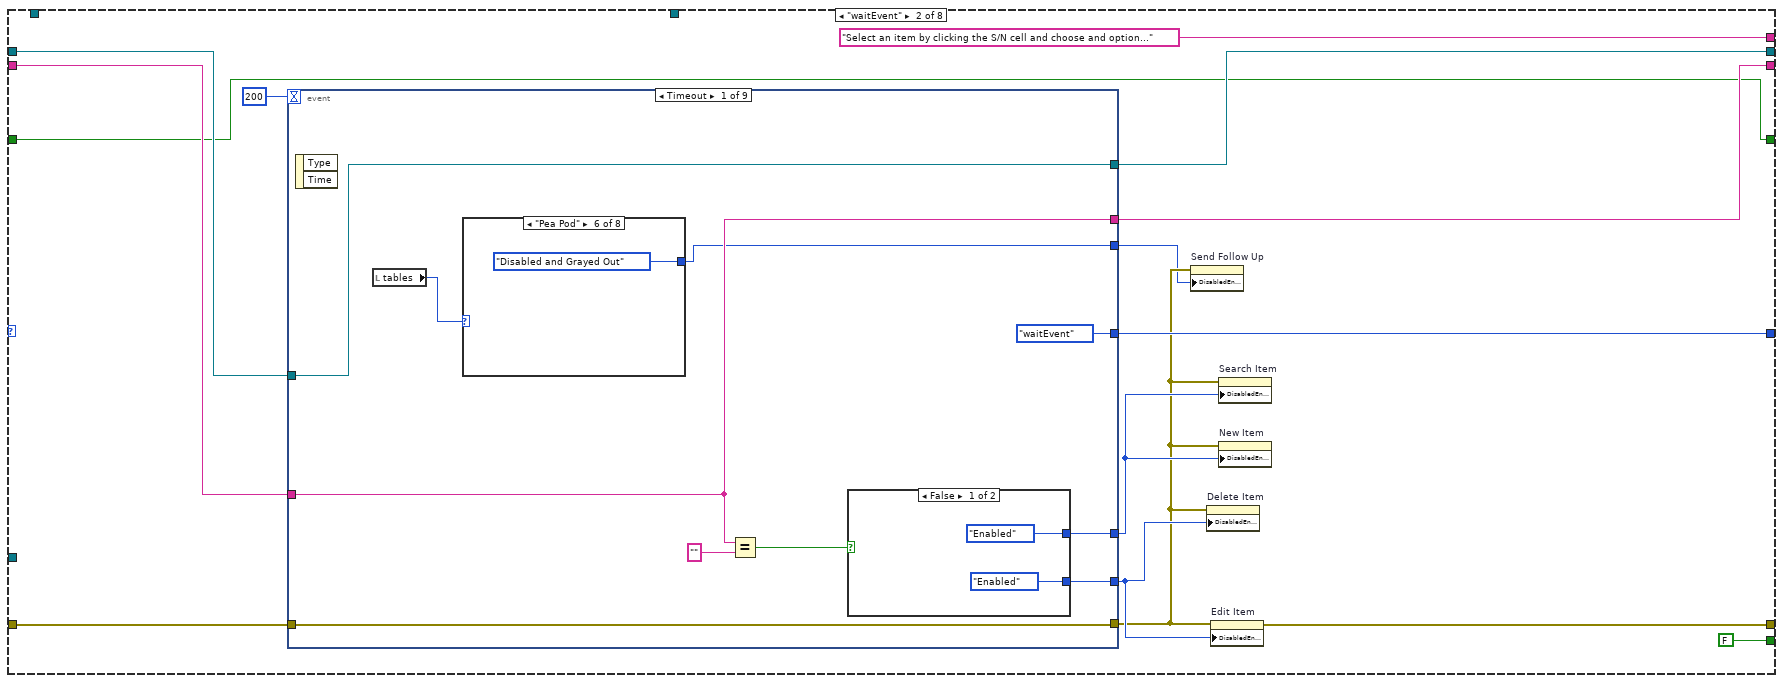
[diagram p3: hidden frame]
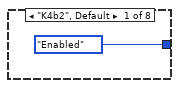
[diagram p4: hidden frame]
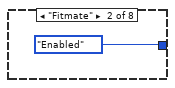
[diagram p5: hidden frame]
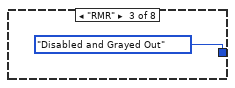
[diagram p6: hidden frame]
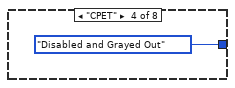
[diagram p7: hidden frame]
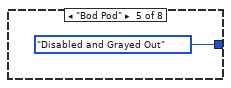
[diagram p8: hidden frame]
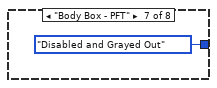
[diagram p9: hidden frame]
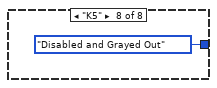
[diagram p10: hidden frame]
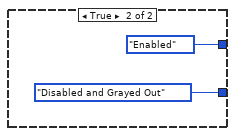
[diagram p11: hidden frame]
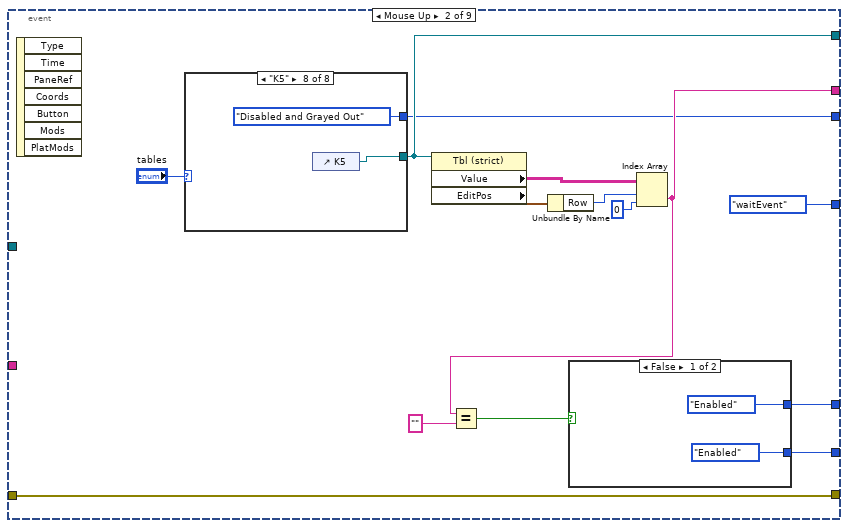
[diagram p12: hidden frame]
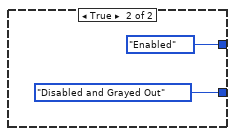
[diagram p13: hidden frame]
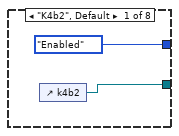
[diagram p14: hidden frame]
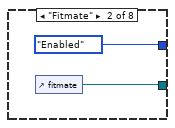
[diagram p15: hidden frame]
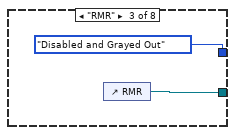
[diagram p16: hidden frame]
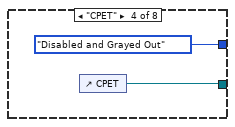
[diagram p17: hidden frame]
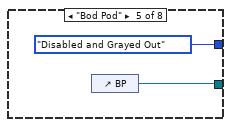
[diagram p18: hidden frame]
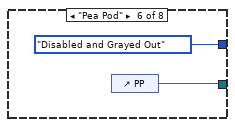
[diagram p19: hidden frame]
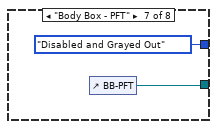
[diagram p20: hidden frame]
diagram:
  n1 = case shown="No Error" "error in (no error)" {
    selector: "error in (no error)" -> [w15 w380]
    tunnel: [w12 w380] -> w3
    tunnel: [w10 w379] -> w1
    tunnel: "reference in" -> [w17 w379]
    frame No Error {
      n2 = call "Project Panels_GetAttributes.vi"("reference in"=w17, "return data? (T)"=FALSE, "error in (no error)"=w15) -> ("reference out"=w10:refnum<class "Project Panels.lvclass">, "attributes ref"=w13:T7, "error out"=w14:errorcluster)  [unwired: 13 in, 1 out]
      n3 = in-place {
        in-place-border: w14 -> [w375]
        in-place-border: [w375] -> w18
        in-place-border: [w374] -> w5
        n4 = in-place-dvr #1(w13) -> (w376:T8)  [unwired: 1 out]
        n5 = in-place {
          in-place-border: [w378] -> w374
          n6 = in-place-cluster #2(w376) -> ("device_controller_ref"=w378:refnum<class "Devices Controller.lvclass">)
          n7 = in-place-cluster #2("device_controller_ref"=w378) -> (w377:T8)
        }
        n8 = in-place-dvr #1(w377) -> (w19:errorcluster)  [unwired: 1 out]
      }
      n9 = Merge Errors(w18, w19) -> (w7:errorcluster)
      n10 = control-ref of="This VI"() -> (w8:refnum<vi>)
      n11 = invoke class="VI" method="Default Vals.Reinit All"(reference=w8, error in=w7) -> ()  [unwired: 1 in, 3 out]
      n12 = control-ref of="K5"() -> (w9:refnum<vi>)
      n13 = while {
        tunnel: w10 -> [w38]
        tunnel: w7 -> [w37]
        tunnel: [w35] -> w12
        shift-right: [w32] -> _
        shift-left: state."initiate" ("state") -> [w36]
        shift-right: [w27] -> _
        shift-left: _ -> [w26]
        shift-right: [w25] -> _
        shift-left: w9 -> [w24]
        tunnel: w10 -> [w23]
        shift-right: [w22] -> _
        shift-left: FALSE ("saved?") -> [w21]
        tunnel: w5 -> [w20]
        stop <- w29 stop-if-true
        n14 = case shown="\"editItem\"" w36 {
          tunnel: w38 -> [w45 _ w226 w248 w277 w295 w337 _]
          tunnel: w37 -> [w41 w109 w228 w247 w275 w298 w336 w352]
          tunnel: [w42 w100 w224 w246 w260 w290 w338 w351] -> w35
          tunnel: [state."waitEvent" ("state") w107 w220 w243 w259 w293 w330 state."stop" ("state")] -> w33
          tunnel: [FALSE FALSE FALSE FALSE FALSE FALSE FALSE TRUE] -> w29
          tunnel: ["Table initialization....." ("title") "Select an item by clicking the S/N cell and choose and option..." ("title") "New Item option selected...." ("title") "Search Item option selected..." ("title") "Edit Item option selected..." ("title") "Send Follow Up option selected" ("title") "Delete Item option selected..." ("title") w357] -> w28
          tunnel: ["" w99 "" "" w268 w294 w333 w360] -> w27
          tunnel: w26 -> [_ w105 _ _ w268 w294 w333 w360]
          tunnel: [w55 w98 w229 w249 w272 w297 w334 w356] -> w25
          tunnel: w24 -> [w55 w101 w229 w249 w272 w297 w334 w356]
          tunnel: w23 -> [w56 _ _ _ _ _ _ _]
          tunnel: [w53 w96 w219 w241 w255 w292 w328 FALSE ("saved?")] -> w22
          tunnel: w21 -> [w53 w96 w216 w239 w253 w292 w326 w350]
          tunnel: w20 -> [_ _ _ _ _ _ _ w349]
          frame "initiate", Default {
            w58 = T4."Disabled and Grayed Out" ("Disabled")
            n15 = property on="K5" class="Tbl (strict)"(error in=w41, "Index Values"=T3 {"Row"=0, "Column"=0}) -> (error out=w40:errorcluster)  [unwired: 1 in, 1 out]
            n16 = call "initiateProducts.vi"("reference in"=w56, "error in (no error)"=w40) -> ("tables"=w54:T9, "error out"=w57:errorcluster)  [unwired: 15 in, 1 out]
            n17 = property on="Search Item" class="Bool"(error in=w57, "DisabledEnum"=w58) -> (error out=w59:errorcluster)  [unwired: 1 in, 1 out]
            n18 = property on="New Item" class="Bool"(error in=w57, "DisabledEnum"=w58) -> (error out=w60:errorcluster)  [unwired: 1 in, 1 out]
            n19 = property on="Edit Item" class="Bool"(error in=w57, "DisabledEnum"=w58) -> (error out=w61:errorcluster)  [unwired: 1 in, 1 out]
            n20 = property on="Send Follow Up" class="Bool"(error in=w57, "DisabledEnum"=w58) -> (error out=w62:errorcluster)  [unwired: 1 in, 1 out]
            n21 = property on="Delete Item" class="Bool"(error in=w57, "DisabledEnum"=w58) -> (error out=w63:errorcluster)  [unwired: 1 in, 1 out]
            n22 = Merge Errors(w59, w60, w61, w62, w63) -> (w64:errorcluster)
            n23 = flat-sequence {
              tunnel: w64 -> [w95]
              tunnel: [w95] -> w50
              frame #0 {
                n24 = local write "statuBar"("Tables initialization....." ("title")) -> ()
              }
            }
            n25 = Unbundle By Name(w54) -> ("k4b2"=→"k4b2":string[][], "fitmate"=→"fitmate":string[][], "RMR"=→"RMR":string[][], "CPET"=→"CPET":string[][], "BP"=→"BP":string[][], "PP"=→"PP":string[][], "k5"=→"K5":string[][], "bb-pft"=→"BB-PFT":string[][])
            n26 = control-ref of="BB-PFT"() -> (w44:refnum<vi>)
            n27 = control-ref of="K5"() -> (w47:refnum<vi>)
            n28 = control-ref of="RMR"() -> (w85:refnum<vi>)
            n29 = control-ref of="k4b2"() -> (w87:refnum<vi>)
            n30 = control-ref of="CPET"() -> (w84:refnum<vi>)
            n31 = control-ref of="BP"() -> (w83:refnum<vi>)
            n32 = control-ref of="PP"() -> (w82:refnum<vi>)
            n33 = control-ref of="fitmate"() -> (w86:refnum<vi>)
            n34 = call "tableCleaner.vi"("error in (no error)"=w50, "K4b2orK5?"=FALSE, "Table in"=w44, "reference in"=w45) -> ("error out"=w48:errorcluster)  [unwired: 6 in, 1 out]
            n35 = call "tableCleaner.vi"("error in (no error)"=w50, "K4b2orK5?"=TRUE, "Table in"=w47, "reference in"=w45) -> ("error out"=w49:errorcluster)  [unwired: 6 in, 1 out]
            n36 = call "tableCleaner.vi"("error in (no error)"=w50, "K4b2orK5?"=FALSE ("K4b2?"), "Table in"=w85, "reference in"=w45) -> ("error out"=w75:errorcluster)  [unwired: 6 in, 1 out]
            n37 = call "tableCleaner.vi"("error in (no error)"=w50, "K4b2orK5?"=FALSE ("K4b2?"), "Table in"=w84, "reference in"=w45) -> ("error out"=w74:errorcluster)  [unwired: 6 in, 1 out]
            n38 = call "tableCleaner.vi"("error in (no error)"=w50, "K4b2orK5?"=FALSE ("K4b2?"), "Table in"=w83, "reference in"=w45) -> ("error out"=w73:errorcluster)  [unwired: 6 in, 1 out]
            n39 = call "tableCleaner.vi"("error in (no error)"=w50, "K4b2orK5?"=FALSE ("K4b2?"), "Table in"=w82, "reference in"=w45) -> ("error out"=w72:errorcluster)  [unwired: 6 in, 1 out]
            n40 = call "tableCleaner.vi"("error in (no error)"=w50, "K4b2orK5?"=FALSE ("K4b2?"), "Table in"=w86, "reference in"=w45) -> ("error out"=w71:errorcluster)  [unwired: 6 in, 1 out]
            n41 = call "tableCleaner.vi"("error in (no error)"=w50, "K4b2orK5?"=TRUE ("K4b2?"), "Table in"=w87, "reference in"=w45) -> ("error out"=w70:errorcluster)  [unwired: 6 in, 1 out]
            n42 = Merge Errors(w48, w49, w75, w74, w73, w72, w71, w70) -> (w42:errorcluster)
            "title" <- "Cosmed Asia Pacific - Products in Aussie" ("title")
          }
          frame "waitEvent" {
            n43 = event shown="[0] Timeout" {
              selector: _ -> [_ _ _ _ _ _ _ _ _]
              dyn-events: _ -> [_ _ _ _ _ _ _ _ _]
              timeout: 200 -> [_ _ _ _ _ _ _ _ _]
              tunnel: w109 -> [w120 w146 w171 w177 w191 w196 w201 w208 w213]
              tunnel: [w120 w146 w171 w177 w191 w196 w201 w208 w213] -> w102
              tunnel: [state."waitEvent" ("state") state."waitEvent" ("state") state."newItem" ("state") state."searchItem" ("state") w179 state."stop" ("state") state."editItem" ("state") state."sendFollowUp" ("state") state."deleteItem" ("state")] -> w107
              tunnel: [w118 w134 w170 w176 w190 w195 w202 w207 w214] -> w104
              tunnel: w105 -> [w113 _ w168 w174 w188 _ w199 w205 w211]
              tunnel: [w115 w135 w170 w176 w190 w195 w202 w207 w214] -> w103
              tunnel: w101 -> [w114 _ w169 w175 w189 w193 w200 w206 w212]
              tunnel: [w113 w136 w168 w174 w188 "" w199 w205 w211] -> w99
              tunnel: [w114 w140 w169 w175 w189 w193 w200 w206 w212] -> w98
              tunnel: [w111 w133 T4."Disabled and Grayed Out" ("Disabled") T4."Disabled and Grayed Out" ("Disabled") T4."Disabled and Grayed Out" ("Disabled") T4."Disabled and Grayed Out" ("Disabled") T4."Disabled and Grayed Out" ("Disabled") T4."Disabled and Grayed Out" ("Disabled") T4."Disabled and Grayed Out" ("Disabled")] -> w97
              event Timeout {
                n44 = event-data() -> ()  [unwired: 1 in, 2 out]
                n45 = local read "tables"() -> (w112:T1)
                n46 = case shown="\"Pea Pod\"" w112 {
                  tunnel: [T4."Enabled" ("Disabled") T4."Enabled" ("Disabled") T4."Disabled and Grayed Out" ("Disabled") T4."Disabled and Grayed Out" ("Disabled") T4."Disabled and Grayed Out" ("Disabled") T4."Disabled and Grayed Out" ("Disabled") T4."Disabled and Grayed Out" ("Disabled") T4."Disabled and Grayed Out" ("Disabled")] -> w111
                  frame "K4b2", Default {
                  }
                  frame "Fitmate" {
                  }
                  frame "RMR" {
                  }
                  frame "CPET" {
                  }
                  frame "Bod Pod" {
                  }
                  frame "Pea Pod" {
                  }
                  frame "Body Box - PFT" {
                  }
                  frame "K5" {
                  }
                }
                n47 = Equal?(x=w113, y="") -> (x = y?=w117:bool)
                n48 = case shown="False" w117 {
                  tunnel: [T4."Enabled" ("Disabled") T4."Disabled and Grayed Out" ("Disabled")] -> w118
                  tunnel: [T4."Enabled" ("Disabled") T4."Enabled" ("Disabled")] -> w115
                  frame False {
                  }
                  frame True {
                  }
                }
              }
              event Mouse Up {
                n49 = event-data() -> ()  [unwired: 1 in, 7 out]
                n50 = case shown="\"K5\"" "tables" {
                  tunnel: [w152 w154 w156 w158 w160 w162 w163 w165] -> w140
                  tunnel: [T4."Enabled" ("Disabled") T4."Enabled" ("Disabled") T4."Disabled and Grayed Out" ("Disabled") T4."Disabled and Grayed Out" ("Disabled") T4."Disabled and Grayed Out" ("Disabled") T4."Disabled and Grayed Out" ("Disabled") T4."Disabled and Grayed Out" ("Disabled") T4."Disabled and Grayed Out" ("Disabled")] -> w133
                  frame "K4b2", Default {
                    n51 = control-ref of="k4b2"() -> (w152:refnum<vi>)
                  }
                  frame "Fitmate" {
                    n52 = control-ref of="fitmate"() -> (w154:refnum<vi>)
                  }
                  frame "RMR" {
                    n53 = control-ref of="RMR"() -> (w156:refnum<vi>)
                  }
                  frame "CPET" {
                    n54 = control-ref of="CPET"() -> (w158:refnum<vi>)
                  }
                  frame "Bod Pod" {
                    n55 = control-ref of="BP"() -> (w160:refnum<vi>)
                  }
                  frame "Pea Pod" {
                    n56 = control-ref of="PP"() -> (w162:refnum<vi>)
                  }
                  frame "Body Box - PFT" {
                    n57 = control-ref of="BB-PFT"() -> (w163:refnum<vi>)
                  }
                  frame "K5" {
                    n58 = control-ref of="K5"() -> (w165:refnum<vi>)
                  }
                }
                n59 = property on="Property Node" class="Tbl (strict)"(reference=w140) -> ("Value"=w144:string[][], "EditPos"=w145:T6)  [unwired: 1 in, 2 out]
                n60 = Unbundle By Name(w145) -> ("Row"=w142:i32)
                n61 = Index Array(array=w144, index (row)=w142, index (col)=0 ("disabled index (col)")) -> (element=w136:string)
                n62 = Equal?(x=w136, y="") -> (x = y?=w138:bool)
                n63 = case shown="False" w138 {
                  tunnel: [T4."Enabled" ("Disabled") T4."Disabled and Grayed Out" ("Disabled")] -> w134
                  tunnel: [T4."Enabled" ("Disabled") T4."Enabled" ("Disabled")] -> w135
                  frame False {
                  }
                  frame True {
                  }
                }
              }
              event "New Item": Mouse Up {
                w170 = T4."Disabled and Grayed Out" ("Disabled")
                n64 = event-data() -> ()  [unwired: 1 in, 7 out]
              }
              event "Search Item": Mouse Up {
                w176 = T4."Disabled and Grayed Out" ("Disabled")
                n65 = event-data() -> ()  [unwired: 1 in, 7 out]
              }
              event Key Down? {
                w190 = T4."Disabled and Grayed Out" ("Disabled")
                n66 = event-data() -> ("Char"=w182:i16)  [unwired: 1 in, 9 out]
                n67 = To Unsigned Byte Integer(number=w182) -> (unsigned 8bit integer=w186:u8)
                n68 = Type Cast(x=w186) -> (*(type *) &x=w185:string)  [unwired: 1 in]
                n69 = Equal?(x=w185, y="f") -> (x = y?=w183:bool)
                n70 = Select(t=state."searchItem" ("state"), s=w183, f=state."waitEvent" ("state")) -> (s? t:f=w179:T2)
                n71 = event-data() -> ()  [unwired: 2 in, 1 out]
              }
              event "Stop Button": Mouse Up {
                w195 = T4."Disabled and Grayed Out" ("Disabled")
                n72 = event-data() -> ()  [unwired: 1 in, 7 out]
              }
              event "Edit Item": Mouse Up {
                w202 = T4."Disabled and Grayed Out" ("Disabled")
                n73 = event-data() -> ()  [unwired: 1 in, 7 out]
              }
              event "Send Follow Up": Mouse Up {
                w207 = T4."Disabled and Grayed Out" ("Disabled")
                n74 = event-data() -> ()  [unwired: 1 in, 7 out]
              }
              event "Delete Item": Mouse Up {
                w214 = T4."Disabled and Grayed Out" ("Disabled")
                n75 = event-data() -> ()  [unwired: 1 in, 7 out]
              }
            }
            n76 = property on="Send Follow Up" class="Bool"(error in=w102, "DisabledEnum"=w97) -> ()  [unwired: 1 in, 2 out]
            n77 = property on="Delete Item" class="Bool"(error in=w102, "DisabledEnum"=w104) -> ()  [unwired: 1 in, 2 out]
            n78 = property on="Edit Item" class="Bool"(error in=w102, "DisabledEnum"=w104) -> (error out=w100:errorcluster)  [unwired: 1 in, 1 out]
            n79 = property on="Search Item" class="Bool"(error in=w102, "DisabledEnum"=w103) -> ()  [unwired: 1 in, 2 out]
            n80 = property on="New Item" class="Bool"(error in=w102, "DisabledEnum"=w103) -> ()  [unwired: 1 in, 2 out]
          }
          frame "newItem" {
            n81 = property class="Tbl (strict)"(reference=w229, error in=w228) -> (error out=w225:errorcluster, "Label.Text"=w227:string)  [unwired: 1 out]
            n82 = case shown="\"fitmate\"" w227 {
              tunnel: [deviceType."rmr" ("deviceType") deviceType."fitmate" ("deviceType") deviceType."bodyBoxPft" ("deviceType") deviceType."bp" ("deviceType") deviceType."cpet" ("deviceType") deviceType."k4b2" ("deviceType")] -> w223
              frame "RMR", Default {
              }
              frame "fitmate" {
              }
              frame "BP" {
              }
              frame "PP" {
              }
              frame "CPET" {
              }
              frame "k4b2" {
              }
            }
            n83 = call "newDevice.vi"("error in (no error)"=w225, "Device Type"=w223, "reference in"=w226) -> ("error out"=w224:errorcluster, "saved?"=w217:bool)  [unwired: 6 in, 1 out]
            n84 = Select(t=TRUE ("saved?"), s=w216, f=w217) -> (s? t:f=w219:bool)
            n85 = Select(t=state."initiate" ("state"), s=w217, f=state."waitEvent" ("state")) -> (s? t:f=w220:T2)
          }
          frame "searchItem" {
            n86 = call "searchEditDevice.vi"("error in (no error)"=w247, "reference in"=w248) -> ("error out"=w246:errorcluster, "saved?"=w240:bool)  [unwired: 7 in, 1 out]
            n87 = Select(t=TRUE ("saved?"), s=w239, f=w240) -> (s? t:f=w241:bool)
            n88 = Select(t=state."initiate" ("state"), s=w240, f=state."waitEvent" ("state")) -> (s? t:f=w243:T2)
          }
          frame "editItem" {
            n89 = property class="Tbl (strict)"(reference=w272, error in=w275) -> (error out=w274:errorcluster, "Label.Text"=w276:string)  [unwired: 1 out]
            n90 = case shown="\"PP\"" w276 {
              tunnel: [deviceType."rmr" ("deviceType") deviceType."k5" ("deviceType") deviceType."bodyBoxPft" ("deviceType") deviceType."fitmate" ("deviceType") deviceType."bp" ("deviceType") deviceType."pp" ("deviceType") deviceType."cpet" ("deviceType") deviceType."k4b2" ("deviceType")] -> w273
              frame "RMR", Default {
              }
              frame "K5" {
              }
              frame "BB-PFT" {
              }
              frame "fitmate" {
              }
              frame "BP" {
              }
              frame "PP" {
              }
              frame "CPET" {
              }
              frame "k4b2" {
              }
            }
            n91 = call "editDevice.vi"("error in (no error)"=w274, "S/N IN"=w268, "Device Type In"=w273, "reference in"=w277) -> ("error out"=w261:errorcluster, "saved?"=w254:bool)  [unwired: 5 in, 1 out]
            n92 = property on="Property Node" class="Tbl (strict)"(reference=w272, error in=w261) -> (reference out=w267:refnum<vi>, error out=w262:errorcluster, "Value"=w271:string[][])
            n93 = Index Array(array=w271, index (col)=0 ("disabled index (col)")) -> (element=w269:string[])  [unwired: 1 in]
            n94 = Search 1D Array(1D array=w269, element=w268) -> (index of element=w264:i32)  [unwired: 1 in]
            n95 = Bundle By Name(cluster=T6 {"Row"=0, "Column"=0} ("Active Cell:Active Cell"), "Row"=w264, "Column"=0) -> (w265:T6)
            n96 = property on="Property Node" class="Tbl (strict)"(reference=w267, error in=w262, "Index Values"=w265) -> (error out=w260:errorcluster)  [unwired: 1 out]
            n97 = Select(t=TRUE ("saved?"), s=w253, f=w254) -> (s? t:f=w255:bool)
            n98 = Select(t=state."initiate" ("state"), s=w254, f=state."waitEvent" ("state")) -> (s? t:f=w259:T2)
          }
          frame "sendFollowUp" {
            n99 = property class="Tbl (strict)"(reference=w297, error in=w298) -> (error out=w296:errorcluster, "Label.Text"=w289:string)  [unwired: 1 out]
            n100 = case shown="\"K5\"" w289 {
              tunnel: [deviceType."rmr" ("deviceType") deviceType."k5" ("deviceType") deviceType."bodyBoxPft" ("deviceType") deviceType."fitmate" ("deviceType") deviceType."bodyBoxPft" ("deviceType") deviceType."bp" ("deviceType") deviceType."cpet" ("deviceType") deviceType."k4b2" ("deviceType")] -> w288
              frame "RMR", Default {
              }
              frame "K5" {
              }
              frame "BB-PFT" {
              }
              frame "fitmate" {
              }
              frame "BP" {
              }
              frame "PP" {
              }
              frame "CPET" {
              }
              frame "k4b2" {
              }
            }
            n101 = call "followUpDevice.vi"("error in (no error)"=w296, "S/N"=w294, "Device Type"=w288, "reference in"=w295) -> ("error out"=w291:errorcluster)  [unwired: 6 in, 1 out]
            n102 = case shown="No Error" w291 {
              selector: w291 -> [w309 w322]
              tunnel: [w310 state."waitEvent" ("state")] -> w293
              tunnel: [w309 w320] -> w290
              frame No Error {
                n103 = flat-sequence {
                  tunnel: [w313] -> w310
                  frame #0 {
                    n104 = Two Button Dialog(message="Do you want to update the Follow Up sent Date?", 1:"No" ("F button name (\"Cancel\")"), 2:"Yes" ("T button name (\"OK\")")) -> (T button?=w312:bool)
                    n105 = Select(t=state."editItem", s=w312, f=state."waitEvent" ("state")) -> (s? t:f=w313:T2)
                  }
                }
              }
              frame Error {
                n106 = call <vilib>:"Simple Error Handler.vi"("error in (no error)"=w322) -> ("source out"=w318:string, "error out"=w321:errorcluster)  [unwired: 4 in, 3 out]
                n107 = call <vilib>:"Clear Errors.vi"("error in (no error)"=w321) -> ("error out"=w320:errorcluster)  [unwired: 5 in, 1 out]
                n108 = One Button Dialog(message=w318, button name ("OK")="OK" ("T button name (\"OK\")")) -> ()  [unwired: 1 out]
              }
            }
          }
          frame "deleteItem" {
            n109 = property class="Tbl (strict)"(reference=w334, error in=w336) -> (error out=w335:errorcluster, "Label.Text"=w325:string)  [unwired: 1 out]
            n110 = case shown="\"K5\"" w325 {
              tunnel: [deviceType."rmr" ("deviceType") deviceType."k5" ("deviceType") deviceType."bodyBoxPft" ("deviceType") deviceType."fitmate" ("deviceType") deviceType."bodyBoxPft" ("deviceType") deviceType."bp" ("deviceType") deviceType."cpet" ("deviceType") deviceType."k4b2" ("deviceType")] -> w324
              frame "RMR", Default {
              }
              frame "K5" {
              }
              frame "BB-PFT" {
              }
              frame "fitmate" {
              }
              frame "BP" {
              }
              frame "PP" {
              }
              frame "CPET" {
              }
              frame "k4b2" {
              }
            }
            n111 = call "deleteDevice.vi"("error in (no error)"=w335, "S/N IN"=w333, "Device Type In"=w324, "reference in"=w337) -> ("error out"=w338:errorcluster, "saved?"=w327:bool)  [unwired: 5 in, 1 out]
            n112 = Select(t=TRUE ("saved?"), s=w326, f=w327) -> (s? t:f=w328:bool)
            n113 = Select(t=state."initiate" ("state"), s=w327, f=state."waitEvent" ("state")) -> (s? t:f=w330:T2)
          }
          frame "stop" {
            n114 = case shown="True" w350 {
              tunnel: w352 -> [w363 w366]
              tunnel: [w363 w367] -> w351
              tunnel: w349 -> [_ w364]
              frame False {
              }
              frame True {
                n115 = flat-sequence {
                  tunnel: w366 -> [w368]
                  tunnel: [w368] -> w365
                  frame #0 {
                    n116 = local write "statuBar"("Wait....I'm saving the new data on the excel file" ("statuBar")) -> ()
                  }
                }
                n117 = call "saveData.vi"("error in (no error)"=w365, "reference in"=w364) -> ("error out"=w367:errorcluster)  [unwired: 8 in, 1 out]
              }
            }
            n118 = Unbundle By Name(w351) -> ("status"=w355:bool)
            n119 = Not(x=w355) -> (.not. x?=w354:bool)
            n120 = case shown="True" w355 {
              tunnel: w351 -> [_ w371]
              frame False {
              }
              frame True {
                n121 = Unbundle By Name(w371) -> ("source"=w370:string)
                n122 = Concatenate Strings("An Error occur: " ("message"), w370) -> (w373:string)
                n123 = One Button Dialog(message=w373) -> ()  [unwired: 1 in, 1 out]
              }
            }
            n124 = Select(t="Stoped from User" ("title"), s=w354, f="Stoped for an Error" ("title")) -> (s? t:f=w357:string)
          }
        }
        "statuBar" <- w28
        "Item Selected (S/N):" <- w27
        n125 = Unbundle By Name(w35) -> ("status"=w34:bool)
        n126 = Not(x=w34) -> (.not. x?=w31:bool)
        n127 = Select(t=w33, s=w31, f=state."stop") -> (s? t:f=w32:T2)
      }
    }
    frame Error {
    }
  }
  "error out" <- w3
  "reference out" <- w1
